vi "Save Profile.vi"(6 "Array 2":dbl[](array[numeric]), 9 "Profile Name":string, 10 "Array":dbl[](array[numeric]), 11 "Output":bool) -> (0 "error out":errorcluster)   [LabVIEW 2016]
uses:
  <vilib>/Utility/file.llb/Write Delimited Spreadsheet (DBL).vi
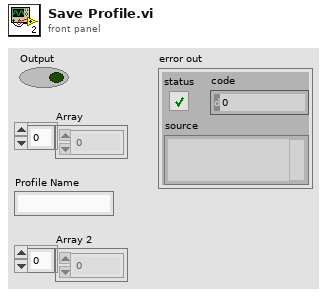
[diagram p1: front panel]
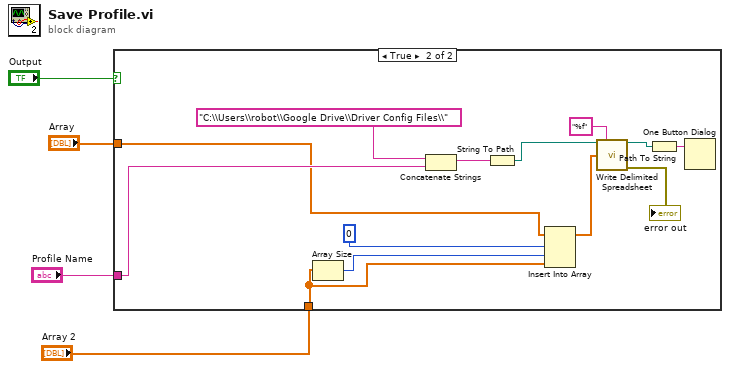
[diagram p0: block diagram]
diagram:
  n1 = case shown="True" "Output" {
    tunnel: "Array" -> [_ w5]
    tunnel: "Array 2" -> [_ w15]
    tunnel: "Profile Name" -> [_ w11]
    frame False {
    }
    frame True {
      n2 = Array Size(array=w15) -> (size(s)=w16:i32)
      n3 = Concatenate Strings("C:\\Users\\robot\\Google Drive\\Driver Config Files\\" ("string"), w11) -> (w10:string)
      n4 = String To Path(string=w10) -> (path=w9:path)
      n5 = Insert Into Array(array=w5, index=0, new element #1=w16, new element #2=w15) -> (w14:dbl[])
      n6 = call-poly <vilib>:"Write Delimited Spreadsheet.vi"("file path (dialog if empty)"=w9, "format (%.3f)"="%f", "1D data"=w14) -> ("new file path (Not A Path if cancelled)"=w7:path, "error out"=→"error out":errorcluster)  [unwired: 11 in]
      n7 = Path To String(path=w7) -> (string=w8:string)
      n8 = One Button Dialog(message=w8) -> ()  [unwired: 1 in, 1 out]
    }
  }
